vi "listDAQsystems.vi"() -> (3 "DAQsystems":string[](array[string]))   [LabVIEW 2022 SP3]
uses:
  Globals/Constants_global.vi
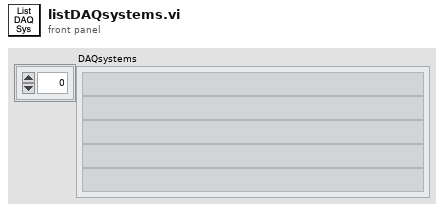
[diagram p1: front panel]
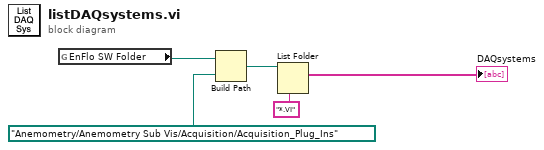
[diagram p0: block diagram]
diagram:
  n1 = global read "Constants_global.vi" "EnFlo SW Folder"() -> (w5:path)
  n2 = Build Path(base path=w5, name or relative path=path "Anemometry/Anemometry Sub Vis/Acquisition/Acquisition_Plug_Ins") -> (appended path=w2:path)
  n3 = List Folder(path=w2, pattern="*.VI") -> (filenames=→"DAQsystems":string[])  [unwired: 2 in, 3 out]
